vi "Test Helper Loop No Time Out Stopping if Error On Launch.vi"(8 "error in (no error)":errorcluster, 11 "Helper Loop Test In":refnum<class "Helper Loop Test.lvclass">) -> (0 "error out":errorcluster, 3 "Helper Loop Test Out":refnum<class "Helper Loop Test.lvclass">)   [LabVIEW 2020, in "Helper Loop Test.lvclass"]
uses:
  Helper Loop Test.lvclass
  C:/Program Files (x86)/National Instruments/LabVIEW 2020/vi.lib/Astemes/LUnit/Test Case.lvclass
  source/Framework Test Suite/Mock Process/Mock Process.lvclass
  C:/Git/astemes-triarc-framework/source/Framework/Process/Process.lvclass
  <vilib>/Astemes/LUnit/Test Case.lvclass/Test Case.ctl
  <vilib>/Astemes/LUnit/LUnit Assertion Result.lvclass/LUnit Assertion Result.ctl
  <vilib>/Astemes/LUnit/LUnit Test Case Result.lvclass/LUnit Test Case Result.ctl
  <vilib>/Astemes/LUnit/LUnit Method Result.lvclass/LUnit Method Result.ctl
  source/Framework/Process/Process.lvclass/Process.ctl
  <vilib>/Astemes/LUnit/Set Assertion Type.vi
  <vilib>/Astemes/LUnit/Palette/Pass.vi
  <vilib>/Astemes/LUnit/Palette/Fail.vi
  source/Framework/Process/Private/SubVIs/Wait for finish.vi
  source/Framework/Process/Protected/Messaging/Enqueue Message.vi
  source/Framework/Process/Private/SubVIs/Set Lifecycle State.vi
  source/Framework/Process/Public/Lifecycle/Get Lifecycle State.vi
  <vilib>/Astemes/LUnit/LUnit Write Assertion Type.vi
  <vilib>/Astemes/LUnit/Add test result.vi
  <vilib>/Astemes/LUnit/LUnit Write Passed.vi
  <vilib>/Astemes/LUnit/LUnit Write Message.vi
  <vilib>/Astemes/LUnit/LUnit Write Description.vi
  source/Framework/Process/Private/SubVIs/Handle Debug Data.vi
  <vilib>/Utility/error.llb/Clear Errors.vi
  <vilib>/Astemes/LUnit/LUnit Record Assertion Result.vi
  source/Framework/Logging/Log Debug.vi
  <vilib>/AdvancedString/1D String Array to Delimited String.vi
  <vilib>/Utility/High Resolution Relative Seconds.vi
  <vilib>/Astemes/LUnit/LUnit Aggregate Assertion Results.vi
  <vilib>/Astemes/LUnit/Assertion Result/LUnit Read Status.vi
  <vilib>/Astemes/LUnit/LUnit Read Message.vi
  <vilib>/Astemes/LUnit/LUnit Read Description.vi
  <vilib>/Astemes/LUnit/Method Result/LUnit Merge Status.vi
  <vilib>/Astemes/LUnit/LUnit Concatenate result strings.vi
  <vilib>/Utility/error.llb/Error Cluster From Error Code.vi
  source/Framework/Process/Public/Read Name.vi
  <vilib>/Astemes/LUnit/LUnit Assertion Result.lvclass
  source/Framework/Process/Process.lvclass
  Helper Loop Test.lvclass/Helper Loop Test.ctl
  <vilib>/Astemes/LUnit/Test Case.lvclass
panel:
  out "timed out?":bool
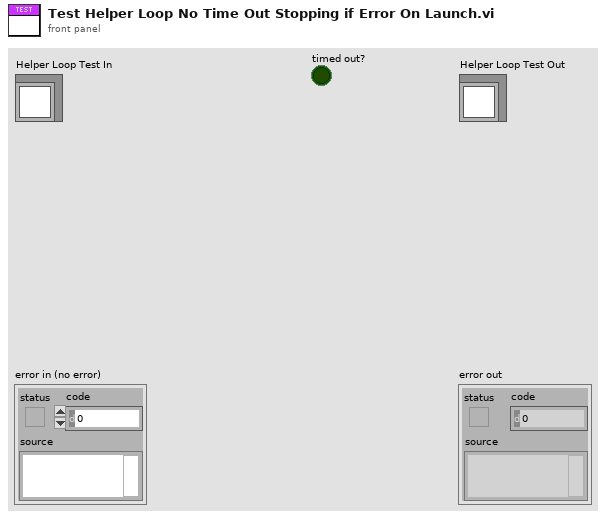
[diagram p1: front panel]
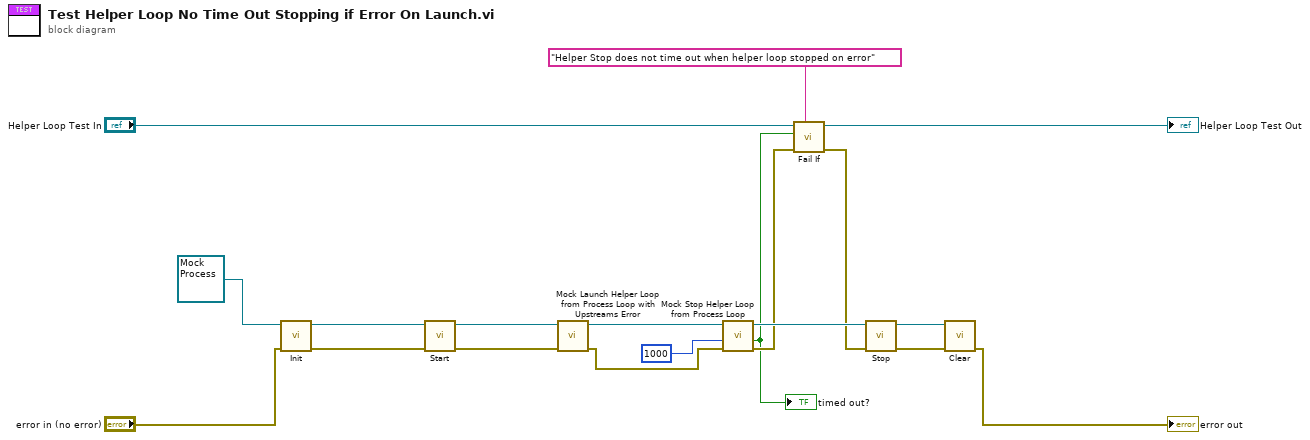
[diagram p0: block diagram]
diagram:
  n1 = call-dynamic "Init.vi"("error in (no error)"="error in (no error)", "Mock Process In"=refnum<class "Mock Process.lvclass"> refnum) -> ("error out"=w18:errorcluster, "Mock Process Out"=w19:refnum<class "Mock Process.lvclass">)  [unwired: 8 in]
  n2 = call "Start.vi"("error in (no error)"=w18, "Process In"=w19) -> ("error out"=w16:errorcluster, "Process Out"=w17:refnum<class "Mock Process.lvclass">)  [unwired: 7 in, 1 out]
  n3 = call "Mock Launch Helper Loop from Process Loop with Upstreams Error.vi"("error in (no error)"=w16, "Mock Process in"=w17) -> ("error out"=w8:errorcluster, "Mock Process out"=w15:refnum<class "Mock Process.lvclass">)  [unwired: 8 in]
  n4 = call "Mock Stop Helper Loop from Process Loop.vi"("error in (no error)"=w8, "timeout in ms (-1)"=1000, "Mock Process in"=w15) -> ("error out"=w13:errorcluster, "timed out?"=w2:bool, "Mock Process out"=w14:refnum<class "Mock Process.lvclass">)  [unwired: 6 in]
  "timed out?" <- w2
  n5 = call <vilib>:"Fail If.vi"("Description"="Helper Stop does not time out when helper loop stopped on error", "error in (no error)"=w13, "Fail?"=w2, "LUnit Test Case In"="Helper Loop Test In") -> ("error out"=w5:errorcluster, "LUnit Test Case Out"=→"Helper Loop Test Out":refnum<class "Helper Loop Test.lvclass">)  [unwired: 6 in]
  n6 = call "Stop.vi"("error in (no error)"=w5, "Process In"=w14) -> ("error out"=w12:errorcluster, "Process Out"=w1:refnum<class "Mock Process.lvclass">)  [unwired: 7 in, 1 out]
  n7 = call-dynamic "Clear.vi"("error in (no error)"=w12, "Mock Process In"=w1) -> ("error out"=→"error out":errorcluster)  [unwired: 9 in]
